vi "数据包.vi"(4 "字符串 6":string, 6 "字符串 5":string, 8 "字符串 4":string, 9 "字符串 3":string, 10 "字符串 2":string, 11 "字符串1":string) -> (3 "连接的字符串":string)   [LabVIEW 2018]
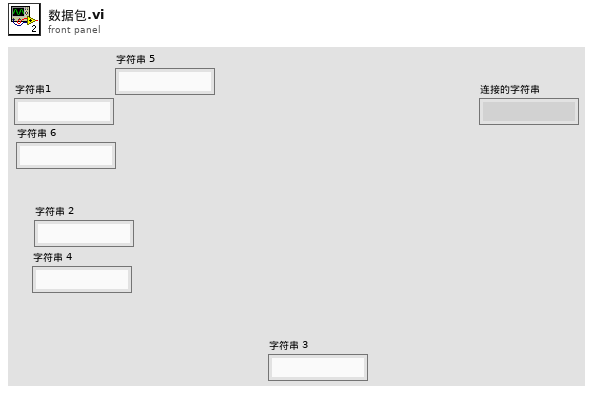
[diagram p1: front panel]
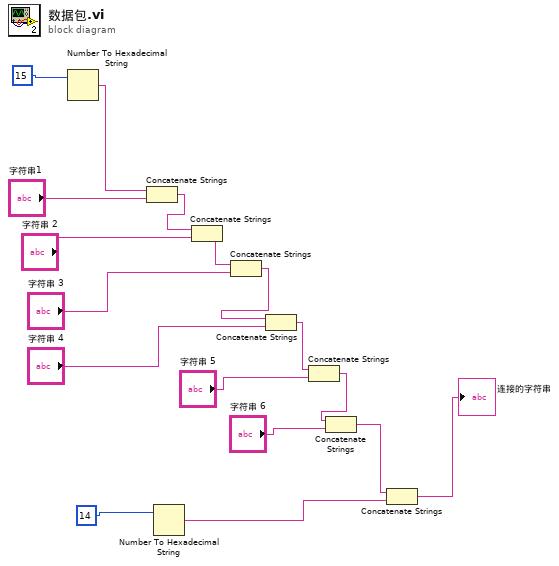
[diagram p0: block diagram]
diagram:
  n1 = Number To Hexadecimal String(2:15) -> (0:w16:string)  [unwired: 1 in]
  n2 = Concatenate Strings(w16, "字符串1") -> (w14:string)
  n3 = Number To Hexadecimal String(2:14) -> (0:w5:string)  [unwired: 1 in]
  n4 = Concatenate Strings(w14, "字符串 2") -> (w12:string)
  n5 = Concatenate Strings(w12, "字符串 3") -> (w9:string)
  n6 = Concatenate Strings(w9, "字符串 4") -> (w7:string)
  n7 = Concatenate Strings(w7, "字符串 5") -> (w3:string)
  n8 = Concatenate Strings(w3, "字符串 6") -> (w1:string)
  n9 = Concatenate Strings(w1, w5) -> (→"连接的字符串":string)
